vi "Periodic Tasks.vi"(8 "error in":errorcluster) -> ()   [LabVIEW 2016]
doc: "This VI runs in parallel to other tasks. It can contain as many user-defined periodic loops as you need. These can carry out PID or other sorts of timed response."
uses:
  <vilib>/platform/TimedLoop/XDataNode/XDataNode.xnode
  <vilib>/Platform/TimedLoop/XDataNode/nitl_modes.ctl
  <vilib>/Platform/TimedLoop/XDataNode/XDNodeRunTimeDep.lvlib
  <vilib>/Platform/TimedLoop/XDataNode/wakeup.ctl
  <vilib>/Platform/TimedLoop/XDataNode/timing_clust.ctl
  MatchTimeNotifications.ctl
  <vilib>/Rock Robotics/WPI/DriverStation/WPI_DriverStationRobotMode2.ctl
  <userlib>/Pneumatics/Support_Code/Pneumatics_Command.ctl
  <vilib>/addons/control/pid/NI_PID_pid.lvlib
  enums/Drive Case Enum.ctl
  <vilib>/addons/control/pid/pid.llb/PID (DBL).vi
  <userlib>/Pneumatics/Support_Code/Pneumatics_Command_Set_Periodic.vi
panel:
  in  "Desired distance":dbl=2.0 format="%#_13g"
  in  "PID gains":T1={"proportional gain (Kc)"=1.0, "integral time (Ti, min)"=0.01, "derivative time (Td, min)"=0.0} {"derivative time (Td, min)" format="%.3f"; "integral time (Ti, min)" format="%.3f"; "proportional gain (Kc)" format="%.3f"}
  in  "GearShift Forward? 2":bool
  in  "Distance":dbl
  in  "PID gains 3":T1={"proportional gain (Kc)"=1.0, "integral time (Ti, min)"=0.01, "derivative time (Td, min)"=0.0} {"derivative time (Td, min)" format="%.3f"; "integral time (Ti, min)" format="%.3f"; "proportional gain (Kc)" format="%.3f"}
  in  "Offset 2":dbl
  in  "Max Throttle 2":dbl
  in  "Negate 2":bool
  in  "PID gains 2":T1={"proportional gain (Kc)"=1.0, "integral time (Ti, min)"=0.01, "derivative time (Td, min)"=0.0} {"derivative time (Td, min)" format="%.3f"; "integral time (Ti, min)" format="%.3f"; "proportional gain (Kc)" format="%.3f"}
  in  "Max Throttle":dbl
  in  "Negate":bool
  in  "Tab Control":enum32{"Drive", "Tab 2"}(tab)
  in  "GearShift Forward?":bool
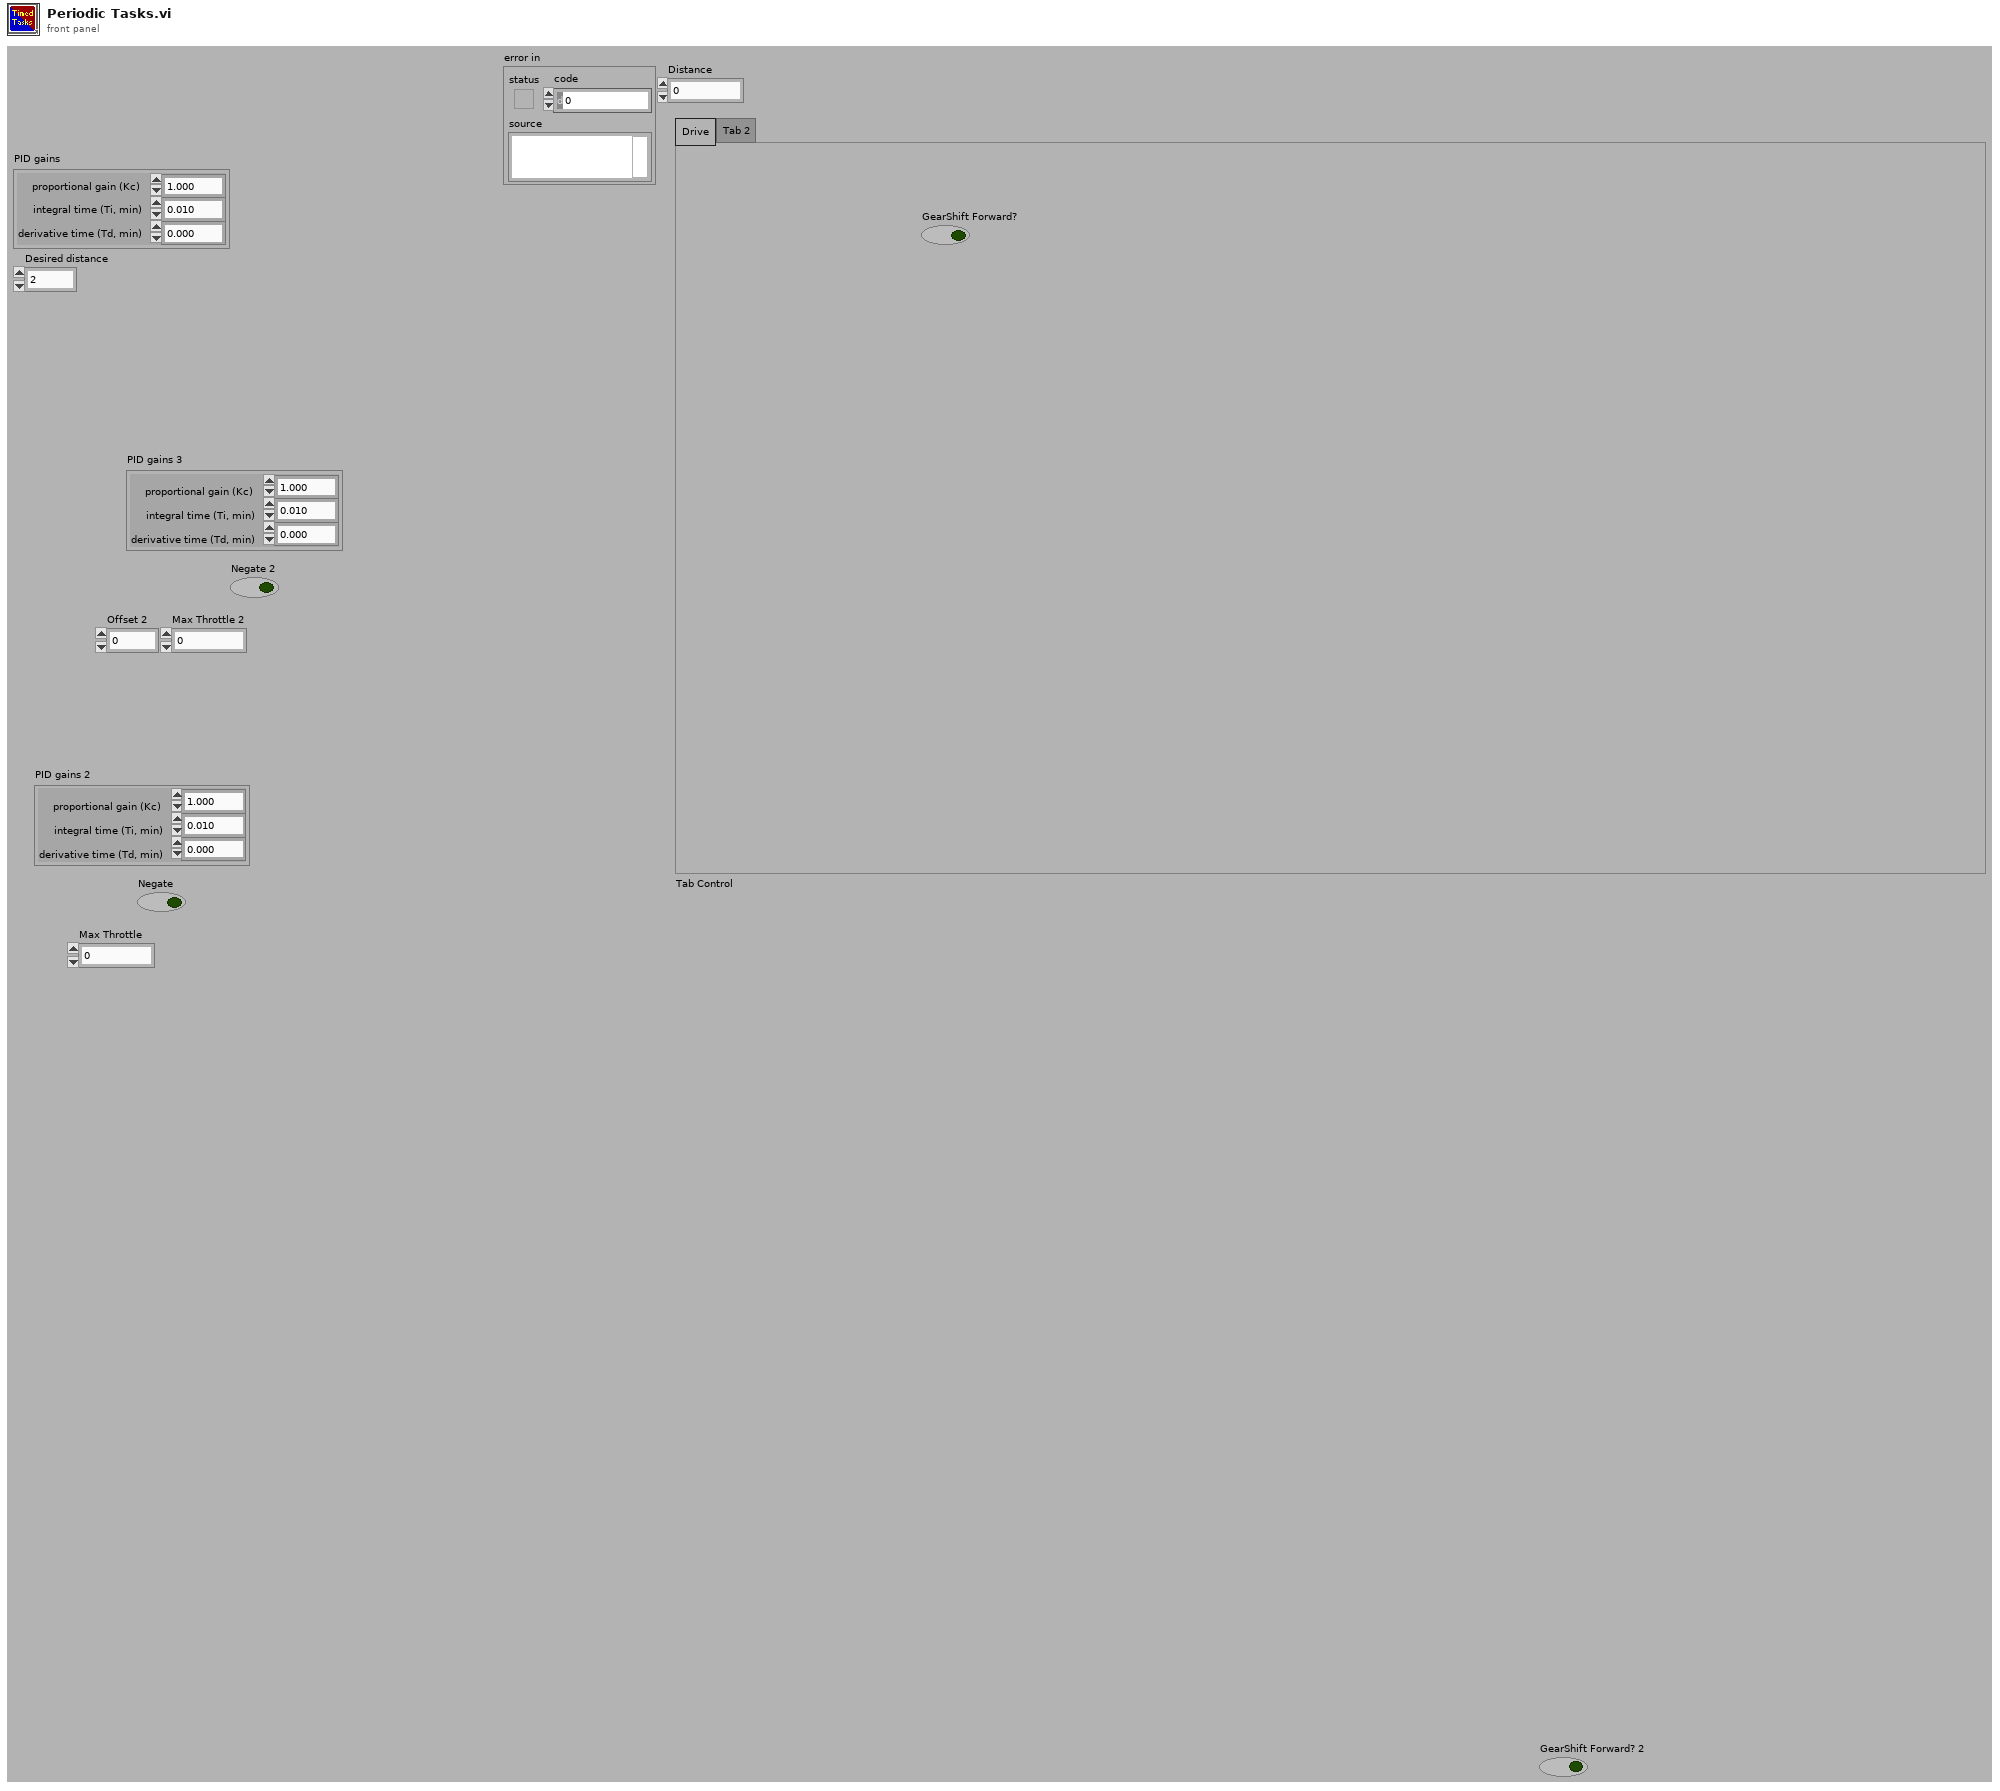
[diagram p1: front panel]
types:
  T1 = cluster{"proportional gain (Kc)":dbl, "integral time (Ti, min)":dbl, "derivative time (Td, min)":dbl}
  T2 = typedef "Drive Case Enum.ctl" = enum16{"Drive", "Gear Approach", "Rope Approach", "Gear Intake"}
  T3 = typedef "MatchTimeNotifications.ctl" = enum16{"oneMinuteLeft", "thirtySecondsLeft", "tenSecondsLeft", "matchOver"}
  T4 = typedef "WPI_SolenoidDevRef.ctl" = cluster{"DevStatus":errorcluster, "Pneumatics Control Module":u8, "Forward Solenoid Channel":T5, "Reverse Solenoid Channel":T5}
  T5 = typedef "WPI_SolenoidChannel.ctl" = enum8{"Solenoid 0", "Solenoid 1", "Solenoid 2", "Solenoid 3", "Solenoid 4", "Solenoid 5", "Solenoid 6", "Solenoid 7", "Invalid"}
  T6 = typedef "Pneumatics_Notifier.ctl" = cluster{"Command":refnum<notifier>, "Status":refnum<queue>}
  T7 = typedef "Solenoid_Control_Loop.ctl" = cluster{"Control Notifier":refnum<notifier>, "Initial Position":T8, "SolenoidDevRef":T4, "Status Loop":refnum<k33>}
  T8 = typedef "Pneumatics_Position.ctl" = enum16{"Forward", "Reverse"}
  T9 = typedef "XDNodeRunTimeDep.lvlib/timing_clust.ctl" = cluster{"Expected End [f-1]":u64, "Actual End [f-1]":u64, "Finished Late? [f-1]":bool, "Expected End [i-1]":u64, "Actual End [i-1]":u64, "Finished Late? [i-1]":bool, "Expected Start [i]":u64, "Actual Start [i]":u64, "Expected Start [f]":u64, "Actual Start [f]":u64, "Source Name":string, "Structure Name":string, "Period":i64, "Deadline":i64, "Offset":i64, "Start":i64, "Priority":i32, "Timeout":i32, "Mode":T10, "Wakeup Reason":T11, "Error":errorcluster, "Source Type":string, "Secondary Source Type":string, "Global End Time":u64, "Global Start Time":u64, "Frame Duration":u64, "Iteration Duration":u64, "Assigned CPU":i32, "I/O Scan Engine Mode":u32}
  T10 = typedef "XDNodeRunTimeDep.lvlib/nitl_modes.ctl" = enum32{"No Change", "Process missed periods, maintain original phase", "Discard missed periods, maintain original phase", "Process missed periods, ignore original phase", "Discard missed periods, ignore original phase"}
  T11 = typedef "XDNodeRunTimeDep.lvlib/wakeup.ctl" = enum32{"Normal", "Aborted", "Asynchronous wakeup", "Timing source error", "Timed loop error", "Timeout"}
  T12 = typedef "Pneumatics_Command.ctl" = enum16{"Nothing", "Forward", "Reverse", "Toggle"}
  T13 = typedef "WPI_DriverStationRobotMode2.ctl" = enum16{"Autonomous Disabled", "Autonomous Enabled", "Teleop Disabled", "Teleop Enabled", "Disconnected", "Finish", "Test Disabled", "Test Enabled", "Emergency Stopped"}
  T14 = typedef "WPI_RobotDriveDevRef.ctl" = cluster{"DevStatus":errorcluster, "Motors[]":T15[], "Square Inputs":bool, "Max Output":dbl}
  T15 = typedef "WPI_MotorControlDeviceRef.ctl" = cluster{"DeviceStatus":errorcluster, "Type":T16, "PWM":cluster{"PWM Channel":T17, "DeadBand":T18}, "CAN":cluster{"Device Number":u8, "SetOutput VI Ref":variant, "GetOutput VI Ref":variant, "Enable VI Ref":variant, "Disable VI Ref":variant, "Data":variant}, "Invert":bool}
  T16 = typedef "WPI_MotorControlType.ctl" = enum16{"PWM", "CAN"}
  T17 = typedef "FPGA_DIOPWMChannel.ctl" = enum8{"PWM 0", "PWM 1", "PWM 2", "PWM 3", "PWM 4", "PWM 5", "PWM 6", "PWM 7", "PWM 8", "PWM 9", "PWM MXP 0", "PWM MXP 1", "PWM MXP 2", "PWM MXP 3", "PWM MXP 4", "PWM MXP 5", "PWM MXP 6", "PWM MXP 7", "PWM MXP 8", "PWM MXP 9", "Invalid"}
  T18 = typedef "WPI_PWMDeadband.ctl" = cluster{"Name":string, "maxPositivePwm":i32, "minPositivePwm":i32, "centerPwm":i32, "maxNegativePwm":i32, "minNegativePwm":i32, "angularRange":u16}
  T19 = typedef "Drive_Code_Bundle.ctl" = cluster{"Sensor Data":T20, "Drive Command rt fifo":refnum<k33>, "Logging Data":refnum<k33>}
  T20 = typedef "Sensor_Cluster.ctl" = cluster{"Gyro Data":cluster{"Gyro RT FIFO":refnum<k33>, "Gyro Current":dbl, "Gyro Hold":dbl}, "Encoder Data":cluster{"Encoder RT FIFO":refnum<k33>, "Encoder Current":dbl, "Encoder Hold":dbl}, "Camera Data":cluster{"Camera RT FIFO":refnum<k33>, "Camera Current":T21}}
  T21 = typedef "Camera_Cluster.ctl" = cluster{" Angle":dbl, "Valid":bool}
  T22 = typedef "WPI_EncoderDevRef.ctl" = cluster{"DevStatus":errorcluster, "EncoderIndex":T23, "CounterIndex":T24, "DistancePerCount":dbl, "Decoding Type":T25}
  T23 = typedef "FPGA_EncoderIdx.ctl" = enum8{"Enc 0", "Enc 1", "Enc 2", "Enc 3", "Enc 4", "Enc 5", "Enc 6", "Enc 7", "Invalid"}
  T24 = typedef "FPGA_CounterCtrSystemIndex.ctl" = enum8{"Ctr 0", "Ctr 1", "Ctr 2", "Ctr 3", "Ctr 4", "Ctr 5", "Ctr 6", "Ctr 7", "Invalid"}
  T25 = typedef "WPI_EncoderType.ctl" = enum16{"1x", "2x", "4x"}
  T26 = typedef "WPI_I2CDevRef.ctl" = cluster{"DevStatus":errorcluster, "Device Address":u8, "Handle":i32, "I2C Bus":T27}
  T27 = typedef "i2c_bus.ctl" = enum16{"I2C On-Board", "I2C MXP", "Invalid"}
  T28 = cluster{"Yaw":dbl, "Roll":dbl, "Pitch":dbl, "Yaw Wind":dbl}
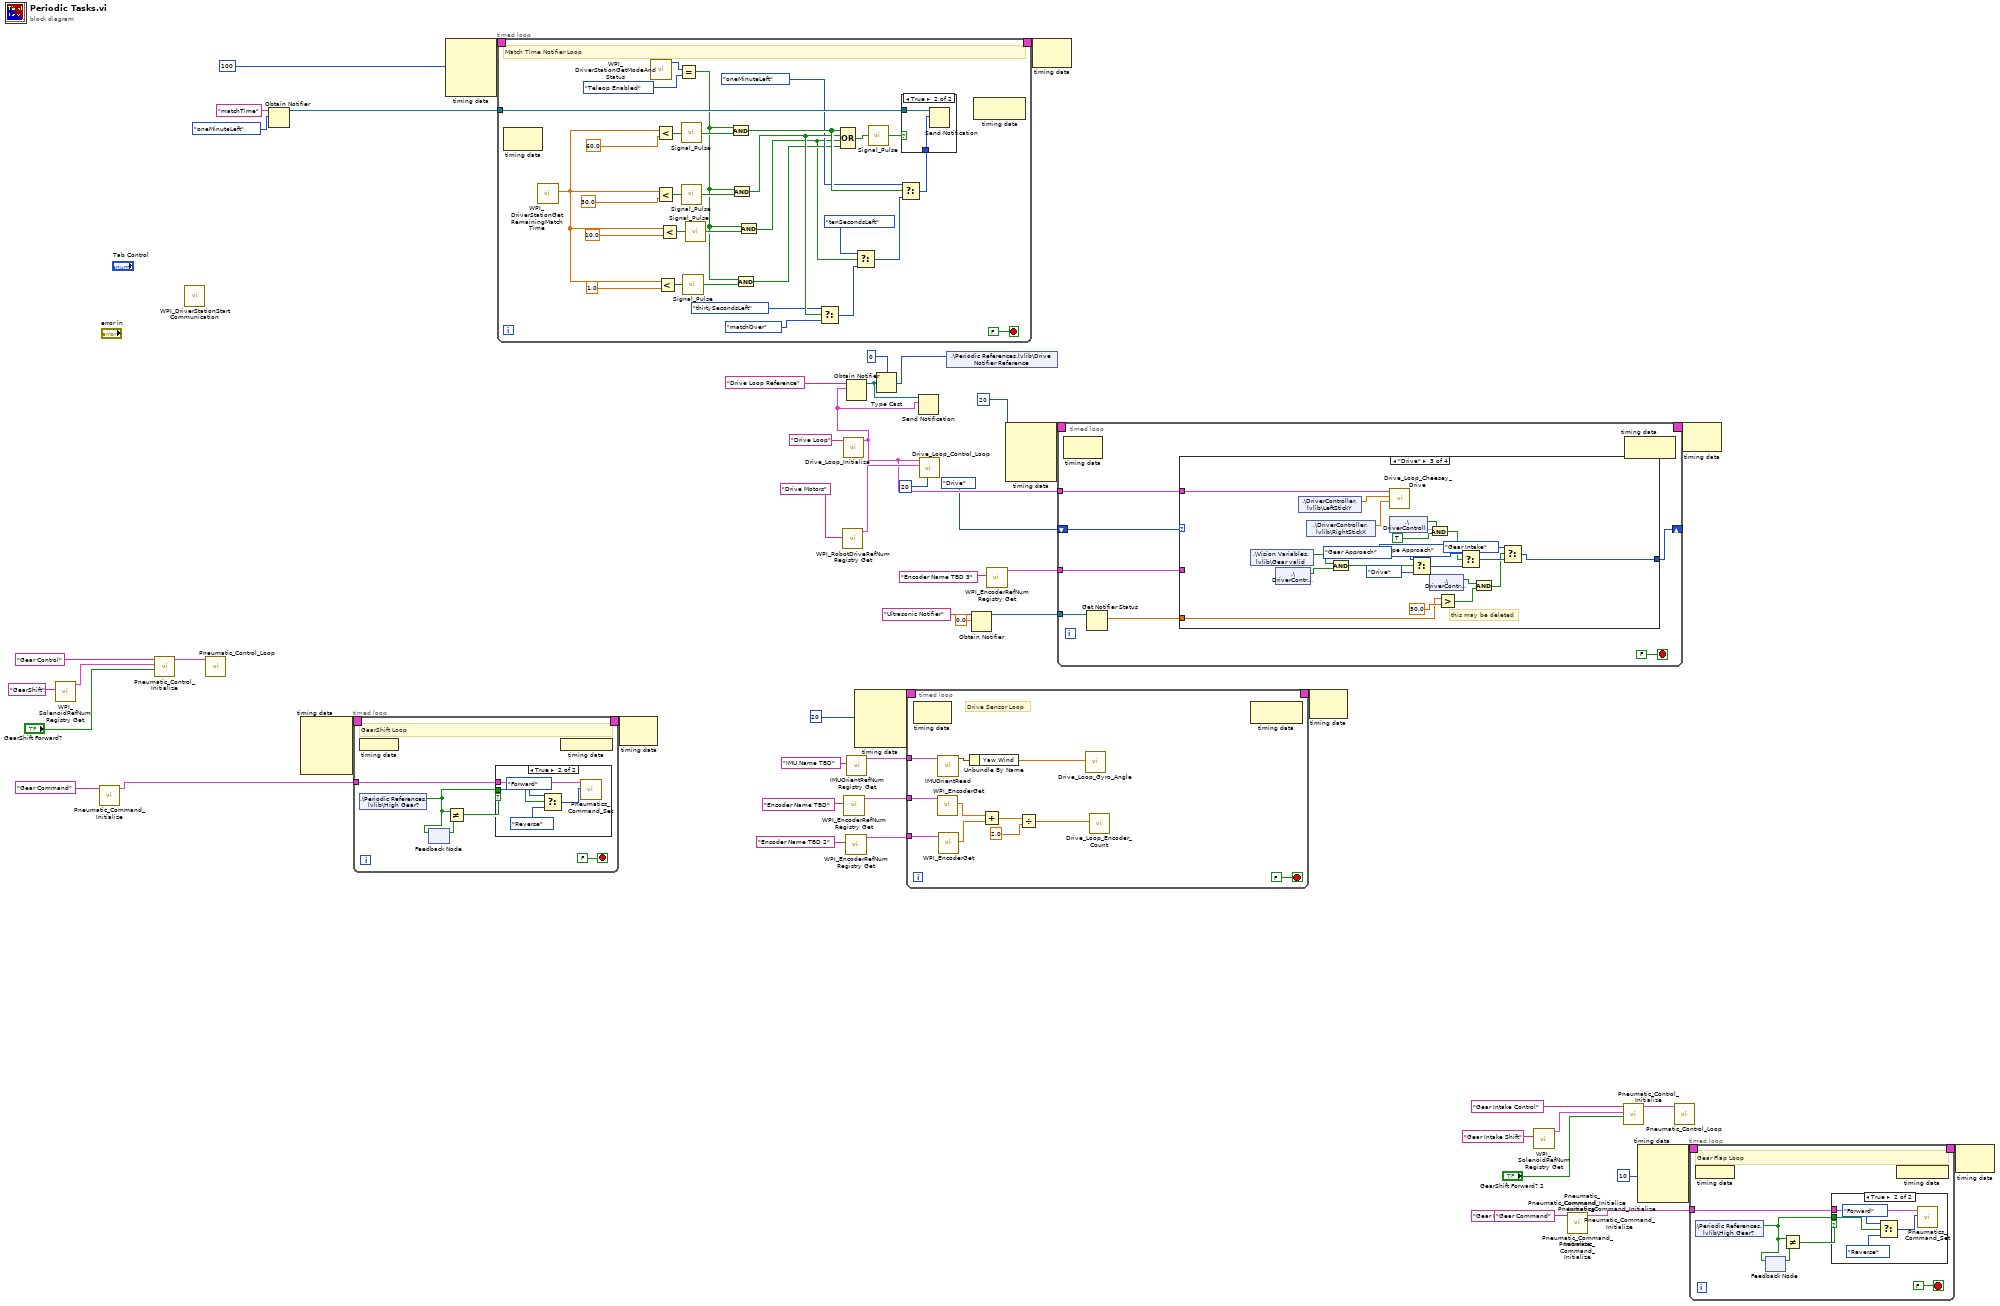
[diagram p0: block diagram]
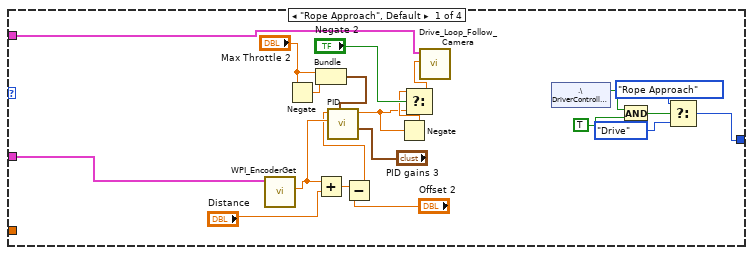
[diagram p2: hidden frame]
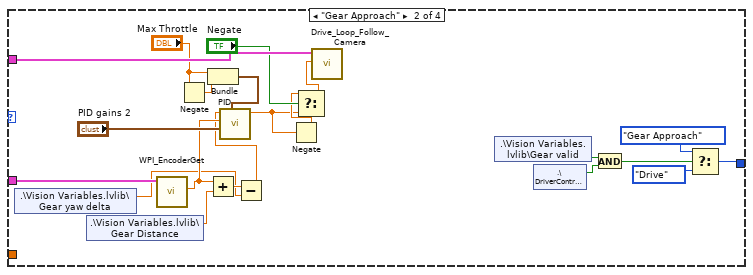
[diagram p3: hidden frame]
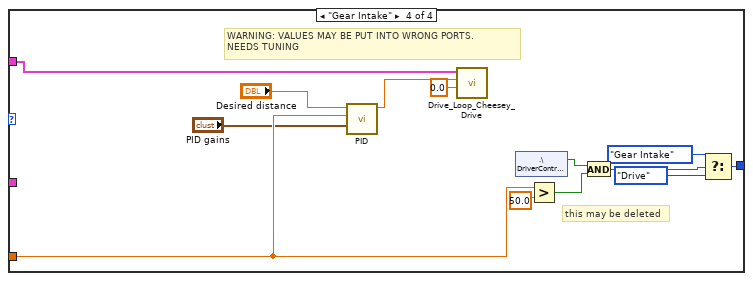
[diagram p4: hidden frame]
diagram:
  n1 = call <vilib>:"WPI_SolenoidRefNum Registry Get.vi"("refnum name"="GearShift") -> ("SolenoidDevRef"=w46:T4)  [unwired: 9 in, 1 out]
  n2 = call <userlib>:"Pneumatic_Command_Initialize.vi"("name (unnamed)"="Gear Command") -> ("Pneumatic Command Cluster"=w29:T6)  [unwired: 9 in, 1 out]
  n3 = call <userlib>:"Pneumatic_Control_Initialize.vi"("Forward?"="GearShift Forward?", "SolenoidDevRef"=w46, "name (unnamed)"="Gear Control" ("Gearshift Control")) -> ("Control Loop"=w50:T7)  [unwired: 7 in, 1 out]
  n4 = call <vilib>:"WPI_DriverStationStart Communication.vi"() -> ()  [unwired: 12 in]
  n5 = call <userlib>:"Pneumatic_Control_Loop.vi"("Cluster in"=w50) -> ()  [unwired: 11 in]
  n6 = Obtain Notifier(name (unnamed)="matchTime", notification data type=MatchTimeNotifications."oneMinuteLeft") -> (notifier out=w53:refnum<notifier>)  [unwired: 2 in, 2 out]
  n7 = node-c288() -> (w49:T9)  [unwired: 4 in]
  n8 = timed-loop {
    timing: w49 -> [_]
    timing-out: [_] -> w48
    tunnel: w29 -> [w61]
    stop <- FALSE stop-if-true
    # "GearShift Loop"
    n9 = node-c288() -> ()  [unwired: 1 in]
    n10 = shared-variable ".\\Periodic References.lvlib\\High Gear?"() -> (w58:bool)  [unwired: 1 in, 1 out]
    n11 = feedback-in #1(w58) -> ()
    n12 = feedback #1() -> (w60:bool)  [unwired: 1 in]
    n13 = Not Equal?(x=w58, y=w60) -> (x != y?=w59:bool)
    n14 = case shown="True" w59 {
      tunnel: w61 -> [_ w67]
      tunnel: w58 -> [_ w66]
      frame False {
      }
      frame True {
        n15 = Select(t=Pneumatics_Command."Forward" ("Solenoid Command"), s=w66, f=Pneumatics_Command."Reverse" ("Solenoid Command")) -> (s? t:f=w63:T12)
        n16 = call-poly <userlib>:"Pneumatics_Command_Set.vi"("Solenoid Command"=w63, "Cluster"=w67) -> ()  [unwired: 9 in, 1 out]
      }
    }
    n17 = node-c288() -> ()  [unwired: 1 out]
  }
  n18 = node-c288(i64 100 ("Period")) -> (w57:T9)  [unwired: 3 in]
  n19 = timed-loop {
    timing: w57 -> [_]
    timing-out: [_] -> w56
    tunnel: w53 -> [w98]
    stop <- FALSE stop-if-true
    # "Match Time Notifier Loop"
    n20 = node-c288() -> ()  [unwired: 1 in, 1 out]
    n21 = call <vilib>:"WPI_DriverStationGetRemainingMatchTime.vi"() -> ("Match Time(s)"=w76:sgl)  [unwired: 10 in, 1 out]
    n22 = call <vilib>:"WPI_DriverStationGetModeAndStatus.vi"() -> ("Robot Mode"=w100:T13)  [unwired: 10 in, 1 out]
    n23 = Less?(x=w76, y=sgl 60.0) -> (x < y?=w93:bool)
    n24 = Less?(x=w76, y=sgl 30.0) -> (x < y?=w97:bool)
    n25 = Less?(x=w76, y=sgl 1.0) -> (x < y?=w89:bool)
    n26 = Less?(x=w76, y=sgl 10.0) -> (x < y?=w78:bool)
    n27 = Equal?(x=w100, y=WPI_DriverStationRobotMode2."Teleop Enabled") -> (x = y?=w75:bool)
    n28 = call <userlib>:"Signal_Pulse.vi"("Input"=w93) -> ("Output"=w87:bool)
    n29 = call <userlib>:"Signal_Pulse.vi"("Input"=w97) -> ("Output"=w96:bool)
    n30 = call <userlib>:"Signal_Pulse.vi"("Input"=w89) -> ("Output"=w88:bool)
    n31 = call <userlib>:"Signal_Pulse.vi"("Input"=w78) -> ("Output"=w79:bool)
    n32 = And(x=w75, y=w87) -> (x .and. y?=w86:bool)
    n33 = And(x=w75, y=w96) -> (x .and. y?=w85:bool)
    n34 = And(x=w75, y=w88) -> (x .and. y?=w74:bool)
    n35 = And(x=w75, y=w79) -> (x .and. y?=w71:bool)
    n36 = Select(t=MatchTimeNotifications."thirtySecondsLeft", s=w85, f=MatchTimeNotifications."matchOver") -> (s? t:f=w73:T3)
    n37 = Compound Arithmetic op=OR(w86, w85, w71, w74) -> (w92:bool)
    n38 = Select(t=MatchTimeNotifications."tenSecondsLeft", s=w71, f=w73) -> (s? t:f=w72:T3)
    n39 = call <userlib>:"Signal_Pulse.vi"("Input"=w92) -> ("Output"=w80:bool)
    n40 = Select(t=MatchTimeNotifications."oneMinuteLeft", s=w86, f=w72) -> (s? t:f=w81:T3)
    n41 = case shown="True" w80 {
      tunnel: w98 -> [_ w102]
      tunnel: w81 -> [_ w101]
      frame False {
      }
      frame True {
        n42 = Send Notification(notification=w101, notifier=w102) -> ()  [unwired: 1 in, 2 out]
      }
    }
    n43 = node-c288() -> ()  [unwired: 1 in, 1 out]
  }
  n44 = node-c288(w48) -> ()  [unwired: 1 out]
  n45 = call <vilib>:"WPI_RobotDriveRefNum Registry Get.vi"("refnum name"="Drive Motors") -> ("RobotDriveDevRef"=w25:T14)  [unwired: 9 in, 1 out]
  n46 = call <userlib>:"Drive_Loop_Initialize.vi"("Name of drive loop (give it a name!)"="Drive Loop") -> ("Drive Loop Cluster"=w17:T19)  [unwired: 9 in, 1 out]
  n47 = call <vilib>:"WPI_EncoderRefNum Registry Get.vi"("refnum name"="Encoder Name TBD") -> ("EncoderDevRef"=w12:T22)  [unwired: 9 in, 1 out]
  n48 = call <vilib>:"WPI_EncoderRefNum Registry Get.vi"("refnum name"="Encoder Name TBD 2") -> ("EncoderDevRef"=w11:T22)  [unwired: 9 in, 1 out]
  n49 = Obtain Notifier(name (unnamed)="Drive Loop Reference", notification data type=w17) -> (notifier out=w21:refnum<notifier>)  [unwired: 2 in, 2 out]
  n50 = call <userlib>:"IMUOrientRefNum Registry Get.vi"("refnum name"="IMU Name TBD") -> ("I2CDevRef out"=w9:T26)  [unwired: 9 in, 1 out]
  n51 = node-c288(i64 20 ("Period")) -> (w14:T9)  [unwired: 3 in]
  n52 = Type Cast(type=u16 0 ("Drive Notifier Reference"), x=w21) -> (*(type *) &x=w18:u16)
  n53 = timed-loop {
    tunnel: w12 -> [w115]
    tunnel: w11 -> [w114]
    timing: w14 -> [_]
    timing-out: [_] -> w13
    tunnel: w9 -> [w106]
    stop <- FALSE stop-if-true
    # "Drive Sensor Loop"
    n54 = node-c288() -> ()  [unwired: 1 in, 1 out]
    n55 = call <vilib>:"WPI_EncoderGet.vi"("EncoderDevRef"=w115) -> ("Distance"=w113:dbl)  [unwired: 5 in, 5 out]
    n56 = call <userlib>:"IMUOrientRead.vi"("I2CDevRef"=w106) -> ("Orient Y/R/P"=w109:T28)  [unwired: 8 in, 6 out]
    n57 = call <vilib>:"WPI_EncoderGet.vi"("EncoderDevRef"=w114) -> ("Distance"=w112:dbl)  [unwired: 5 in, 5 out]
    n58 = Unbundle By Name(w109) -> ("Yaw Wind"=w108:dbl)
    n59 = Add(x=w113, y=w112) -> (x+y=w110:dbl)
    n60 = Divide(x=w110, y=2.0 ("x")) -> (x/y=w105:dbl)
    n61 = call <userlib>:"Drive_Loop_Gyro_Angle.vi"("Yaw Wind"=w108) -> ()  [unwired: 11 in]
    n62 = call <userlib>:"Drive_Loop_Encoder_Count.vi"("Distance"=w105) -> ()  [unwired: 11 in]
    n63 = node-c288() -> ()  [unwired: 1 in, 1 out]
  }
  n64 = Send Notification(notification=w17, notifier=w21) -> ()  [unwired: 1 in, 2 out]
  n65 = call <userlib>:"Drive_Loop_Control_Loop.vi"("Period \n- Amount of time between iterations of the timed control loop"=i64 20 ("Period \n- Amount of time between iterations of the timed control loop"), "RobotDriveDevRef"=w25, "Control Cluster"=w17) -> ()  [unwired: 9 in]
  n66 = shared-variable ".\\Periodic References.lvlib\\Drive Notifier Reference"(w18) -> ()  [unwired: 1 in, 1 out]
  n67 = Obtain Notifier(name (unnamed)="Ultrasonic Notifier", notification data type=0.0) -> (notifier out=w1:refnum<notifier>)  [unwired: 2 in, 2 out]
  n68 = call <vilib>:"WPI_EncoderRefNum Registry Get.vi"("refnum name"="Encoder Name TBD 3") -> ("EncoderDevRef"=w4:T22)  [unwired: 9 in, 1 out]
  n69 = node-c288(i64 20 ("Period")) -> (w27:T9)  [unwired: 3 in]
  n70 = node-c288(w56) -> ()  [unwired: 1 out]
  n71 = timed-loop {
    tunnel: w17 -> [w123]
    timing: w27 -> [_]
    timing-out: [_] -> w26
    shift-right: [w121] -> _
    shift-left: Drive_Case_Enum."Drive" -> [w122]
    tunnel: w4 -> [w120]
    tunnel: w1 -> [w119]
    stop <- FALSE stop-if-true
    n72 = node-c288() -> ()  [unwired: 1 in, 1 out]
    n73 = Get Notifier Status(notifier=w119) -> (current notification=w118:dbl)  [unwired: 1 in, 4 out]
    n74 = case shown="\"Drive\"" w122 {
      tunnel: w123 -> [w128 w168 w187 w192]
      tunnel: [w147 w151 w169 w202] -> w121
      tunnel: w120 -> [w127 w149 _ _]
      tunnel: w118 -> [_ _ w171 w194]
      frame "Rope Approach", Default {
        n75 = call <vilib>:"WPI_EncoderGet.vi"("EncoderDevRef"=w127) -> ("Distance"=w140:dbl)  [unwired: 5 in, 5 out]
        n76 = Negate(x="Max Throttle 2") -> (-x=w135:dbl)
        n77 = Bundle("Max Throttle 2"="Max Throttle 2", w135) -> (w134:cluster{"Max Throttle 2":dbl, dbl})  [unwired: 1 in]
        n78 = Add(x=w140, y="Distance") -> (x+y=w139:dbl)
        n79 = Subtract(x=w139, y="Offset 2") -> (x-y=w137:dbl)
        n80 = call-poly <vilib>:"PID.vi"("output range"=w134, "PID gains"="PID gains 3", "process variable"=w140, "setpoint"=w137) -> ("output"=w131:dbl)  [unwired: 6 in, 1 out]
        n81 = Negate(x=w131) -> (-x=w132:dbl)
        n82 = Select(t=w132, s="Negate 2", f=w131) -> (s? t:f=w130:dbl)
        n83 = call <userlib>:"Drive_Loop_Follow_Camera.vi"("Power Level #6"=w130, "Drive Loop Cluster"=w128) -> ()  [unwired: 10 in]
        n84 = shared-variable ".\\DriverController.lvlib\\RT"() -> (w144:bool)  [unwired: 1 in, 1 out]
        n85 = And(x=w144, y=TRUE) -> (x .and. y?=w142:bool)
        n86 = Select(t=Drive_Case_Enum."Rope Approach", s=w142, f=Drive_Case_Enum."Drive") -> (s? t:f=w147:T2)
      }
      frame "Gear Approach" {
        n87 = shared-variable ".\\Vision Variables.lvlib\\Gear yaw delta"() -> (w148:dbl)  [unwired: 1 in, 1 out]
        n88 = shared-variable ".\\Vision Variables.lvlib\\Gear Distance"() -> (w163:dbl)  [unwired: 1 in, 1 out]
        n89 = call <vilib>:"WPI_EncoderGet.vi"("EncoderDevRef"=w149) -> ("Distance"=w166:dbl)  [unwired: 5 in, 5 out]
        n90 = Negate(x="Max Throttle") -> (-x=w161:dbl)
        n91 = Bundle("Max Throttle"="Max Throttle", w161) -> (w160:cluster{"Max Throttle":dbl, dbl})  [unwired: 1 in]
        n92 = Add(x=w166, y=w163) -> (x+y=w165:dbl)
        n93 = Subtract(x=w165, y=w148) -> (x-y=w164:dbl)
        n94 = call-poly <vilib>:"PID.vi"("output range"=w160, "PID gains"="PID gains 2", "process variable"=w166, "setpoint"=w164) -> ("output"=w157:dbl)  [unwired: 6 in, 1 out]
        n95 = Negate(x=w157) -> (-x=w158:dbl)
        n96 = Select(t=w158, s="Negate", f=w157) -> (s? t:f=w156:dbl)
        n97 = call <userlib>:"Drive_Loop_Follow_Camera.vi"("Power Level #6"=w156, "Drive Loop Cluster"=w168) -> ()  [unwired: 10 in]
        n98 = shared-variable ".\\Vision Variables.lvlib\\Gear valid"() -> (w154:bool)  [unwired: 1 in, 1 out]
        n99 = shared-variable ".\\DriverController.lvlib\\A"() -> (w155:bool)  [unwired: 1 in, 1 out]
        n100 = And(x=w154, y=w155) -> (x .and. y?=w153:bool)
        n101 = Select(t=Drive_Case_Enum."Gear Approach", s=w153, f=Drive_Case_Enum."Drive") -> (s? t:f=w151:T2)
      }
      frame "Drive" {
        # "this may be deleted"
        n102 = shared-variable ".\\Vision Variables.lvlib\\Gear valid"() -> (w185:bool)  [unwired: 1 in, 1 out]
        n103 = shared-variable ".\\DriverController.lvlib\\A"() -> (w186:bool)  [unwired: 1 in, 1 out]
        n104 = shared-variable ".\\DriverController.lvlib\\LeftStickY"() -> (w188:dbl)  [unwired: 1 in, 1 out]
        n105 = shared-variable ".\\DriverController.lvlib\\RightStickX"() -> (w189:dbl)  [unwired: 1 in, 1 out]
        n106 = And(x=w185, y=w186) -> (x .and. y?=w184:bool)
        n107 = shared-variable ".\\DriverController.lvlib\\RT"() -> (w179:bool)  [unwired: 1 in, 1 out]
        n108 = call <userlib>:"Drive_Loop_Cheesey_Drive.vi"("Wheel"=w189, "Throttle"=w188, "Drive Loop Cluster"=w187) -> ()  [unwired: 9 in]
        n109 = Select(t=Drive_Case_Enum."Gear Approach", s=w184, f=Drive_Case_Enum."Drive") -> (s? t:f=w182:T2)
        n110 = And(x=w179, y=TRUE) -> (x .and. y?=w177:bool)
        n111 = shared-variable ".\\DriverController.lvlib\\X"() -> (w174:bool)  [unwired: 1 in, 1 out]
        n112 = Greater?(x=w171, y=50.0) -> (0:w175:bool)
        n113 = Select(t=Drive_Case_Enum."Rope Approach", s=w177, f=w182) -> (s? t:f=w176:T2)
        n114 = And(x=w174, y=w175) -> (x .and. y?=w173:bool)
        n115 = Select(t=Drive_Case_Enum."Gear Intake", s=w173, f=w176) -> (s? t:f=w169:T2)
      }
      frame "Gear Intake" {
        # "WARNING: VALUES MAY BE PUT INTO WRONG PORTS.\nNEEDS TUNING"
        # "this may be deleted"
        n116 = call-poly <vilib>:"PID.vi"("PID gains"="PID gains", "process variable"=w194, "setpoint"="Desired distance") -> ("output"=w191:dbl)  [unwired: 7 in, 1 out]
        n117 = call <userlib>:"Drive_Loop_Cheesey_Drive.vi"("Wheel"=0.0, "Throttle"=w191, "Drive Loop Cluster"=w192) -> ()  [unwired: 9 in]
        n118 = shared-variable ".\\DriverController.lvlib\\X"() -> (w197:bool)  [unwired: 1 in, 1 out]
        n119 = Greater?(x=w194, y=50.0) -> (0:w198:bool)
        n120 = And(x=w197, y=w198) -> (x .and. y?=w199:bool)
        n121 = Select(t=Drive_Case_Enum."Gear Intake", s=w199, f=Drive_Case_Enum."Drive") -> (s? t:f=w202:T2)
      }
    }
    n122 = node-c288() -> ()  [unwired: 1 in, 1 out]
  }
  n123 = node-c288(w13) -> ()  [unwired: 1 out]
  n124 = call <vilib>:"WPI_SolenoidRefNum Registry Get.vi"("refnum name"="Gear Intake Shift") -> ("SolenoidDevRef"=w37:T4)  [unwired: 9 in, 1 out]
  n125 = call <userlib>:"Pneumatic_Command_Initialize.vi"("name (unnamed)"="Gear Intake Command") -> ()  [unwired: 9 in, 2 out]
  n126 = call <userlib>:"Pneumatic_Command_Initialize.vi"("name (unnamed)"="Gear Command") -> ()  [unwired: 9 in, 2 out]
  n127 = call <userlib>:"Pneumatic_Command_Initialize.vi"("name (unnamed)"="Gear Command") -> ()  [unwired: 9 in, 2 out]
  n128 = call <userlib>:"Pneumatic_Command_Initialize.vi"("name (unnamed)"="Gear Command") -> ()  [unwired: 9 in, 2 out]
  n129 = call <userlib>:"Pneumatic_Command_Initialize.vi"("name (unnamed)"="Gear Command") -> ()  [unwired: 9 in, 2 out]
  n130 = call <userlib>:"Pneumatic_Command_Initialize.vi"("name (unnamed)"="Gear Command") -> ("Pneumatic Command Cluster"=w39:T6)  [unwired: 9 in, 1 out]
  n131 = call <userlib>:"Pneumatic_Control_Initialize.vi"("Forward?"="GearShift Forward? 2", "SolenoidDevRef"=w37, "name (unnamed)"="Gear Intake Control" ("Gearshift Control")) -> ("Control Loop"=w41:T7)  [unwired: 7 in, 1 out]
  n132 = node-c288(i64 10 ("Period")) -> (w44:T9)  [unwired: 3 in]
  n133 = call <userlib>:"Pneumatic_Control_Loop.vi"("Cluster in"=w41) -> ()  [unwired: 11 in]
  n134 = node-c288(w26) -> ()  [unwired: 1 out]
  n135 = timed-loop {
    timing: w44 -> [_]
    timing-out: [_] -> w43
    tunnel: w39 -> [w206]
    stop <- FALSE stop-if-true
    # "Gear Flap Loop"
    n136 = node-c288() -> ()  [unwired: 1 in]
    n137 = shared-variable ".\\Periodic References.lvlib\\High Gear?"() -> (w203:bool)  [unwired: 1 in, 1 out]
    n138 = feedback-in #2(w203) -> ()
    n139 = feedback #2() -> (w205:bool)  [unwired: 1 in]
    n140 = Not Equal?(x=w203, y=w205) -> (x != y?=w204:bool)
    n141 = case shown="True" w204 {
      tunnel: w206 -> [_ w212]
      tunnel: w203 -> [_ w211]
      frame False {
      }
      frame True {
        n142 = Select(t=Pneumatics_Command."Forward" ("Solenoid Command"), s=w211, f=Pneumatics_Command."Reverse" ("Solenoid Command")) -> (s? t:f=w208:T12)
        n143 = call-poly <userlib>:"Pneumatics_Command_Set.vi"("Solenoid Command"=w208, "Cluster"=w212) -> ()  [unwired: 9 in, 1 out]
      }
    }
    n144 = node-c288() -> ()  [unwired: 1 out]
  }
  n145 = node-c288(w43) -> ()  [unwired: 1 out]
